vi "Initialize.vi"(8 "error in":errorcluster, 9 "Channels Amount":u8=1, 10 "InstanceName":string, 11 "Climate Chamber Cluster.lvclass":refnum<class "Climate Chamber Cluster.lvclass">) -> (0 "error out":errorcluster, 3 "Climate Chamber Cluster.lvclass out":refnum<class "Climate Chamber Cluster.lvclass">)   [LabVIEW 2023, in "Climate Chamber Cluster.lvclass"]
uses:
  Climate Chamber Cluster.lvclass
  Climate Chamber Cluster.lvclass/Climate Chamber Cluster.ctl
  310450b7-dc98-4d07-9383-43575356c6f4.vi
  702b615c-4a60-4ec7-b760-116075cb0d01.vi
  78d7c854-17cb-40e3-91c7-b55f38b06fec.vi
  34d8de8f-da75-496c-99f7-44cc67c60a3e.vi
  310450b7-dc98-4d07-9383-43575356c6f4.vi/4bc1c15b-36ab-481f-b8dd-c64075ce723a.vi
  702b615c-4a60-4ec7-b760-116075cb0d01.vi/4bc1c15b-36ab-481f-b8dd-c64075ce723a.vi
  78d7c854-17cb-40e3-91c7-b55f38b06fec.vi/4bc1c15b-36ab-481f-b8dd-c64075ce723a.vi
  34d8de8f-da75-496c-99f7-44cc67c60a3e.vi/4bc1c15b-36ab-481f-b8dd-c64075ce723a.vi
  <vilib>/ADAS Replay HIL/AdasHilServices/AdasHilServices Fill In Error Info Ex.vi
  Utilities/Utilities.lvlib
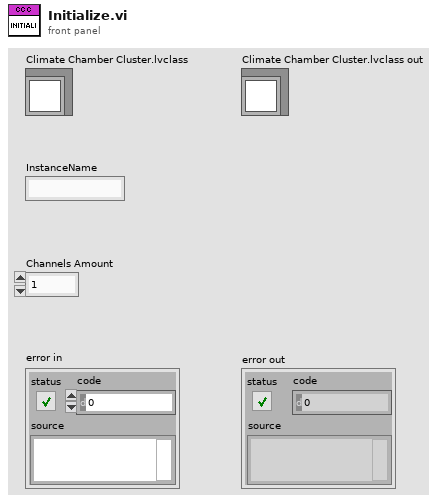
[diagram p1: front panel]
types:
  T1 = cluster{"OnOff.ACT":bool, "ErrorAcknowledge.ACT":bool}
  T2 = cluster{"OnOff.STS":i32, "Error.STS":i32, "Watchdog.STS":i32}
  T3 = cluster{"Temperature.SP":dbl, "TemperatureMIN.SP":dbl, "TemperatureMAX.SP":dbl, "TemperatureGrad.SP":dbl, "Humidity.SP":dbl, "HumidityMIN.SP":dbl, "HumidityMAX.SP":dbl, "HumidityGrad.SP":dbl}[]
  T4 = cluster{"Temperature.AV":dbl, "Humidity.AV":dbl}[]
  T5 = cluster{"Temperature.SP":dbl, "TemperatureMIN.SP":dbl, "TemperatureMAX.SP":dbl, "TemperatureGrad.SP":dbl, "Humidity.SP":dbl, "HumidityMIN.SP":dbl, "HumidityMAX.SP":dbl, "HumidityGrad.SP":dbl}
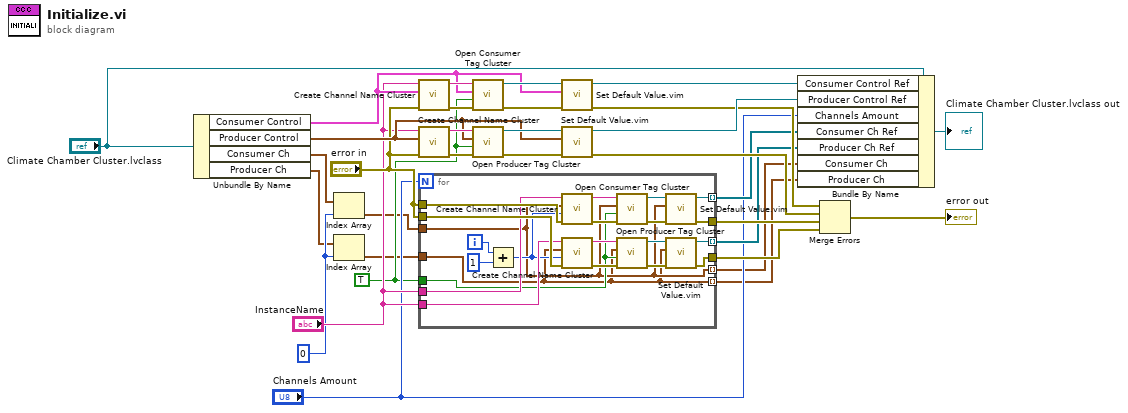
[diagram p0: block diagram]
diagram:
  w5 = 0 ("index")
  w8 = TRUE ("Create if not found? (T)")
  n1 = Unbundle By Name("Climate Chamber Cluster.lvclass") -> ("Consumer Control"=w18:T1, "Producer Control"=w19:T2, "Consumer Ch"=w7:T3, "Producer Ch"=w4:T4)
  n2 = Index Array(array=w7, index=w5) -> (element=w6:T5)
  n3 = Index Array(array=w4, index=w5) -> (element=w3:cluster{"Temperature.AV":dbl, "Humidity.AV":dbl})
  n4 = call "Create Channel Name Cluster.vi"("error in"="error in", "Cluster"=w18, "Instance Name"="InstanceName") -> ("error out"=w23:errorcluster, "Data Channel Name"=w32:string)  [unwired: 7 in]
  n5 = call "Create Channel Name Cluster.vi"("error in"="error in", "Cluster"=w19, "Instance Name"="InstanceName") -> ("error out"=w24:errorcluster, "Data Channel Name"=w31:string)  [unwired: 7 in]
  n6 = for {
    N: "Channels Amount" -> [_]
    tunnel: "error in" -> [w46]
    tunnel: "InstanceName" -> [w45]
    tunnel: "error in" -> [w44]
    tunnel: "InstanceName" -> [w43]
    tunnel: [w42] -> w15
    tunnel: [w41] -> w14
    tunnel: [w40] -> w12 mode=indexing
    tunnel: [w39] -> w11 mode=indexing
    tunnel: w6 -> [w34]
    tunnel: w3 -> [w33]
    tunnel: w8 -> [w38]
    tunnel: [w34] -> w2 mode=indexing
    tunnel: [w33] -> w1 mode=indexing
    i -> [w37]
    n7 = Add(x=w37, y=1) -> (x+y=w36:i32)
    n8 = call "Create Channel Name Cluster.vi"("error in"=w44, "Numeric"=w36, "Cluster"=w34, "Instance Name"=w43) -> ("error out"=w52:errorcluster, "Data Channel Name"=w47:string)  [unwired: 6 in]
    n9 = call "Create Channel Name Cluster.vi"("error in"=w46, "Numeric"=w36, "Cluster"=w33, "Instance Name"=w45) -> ("error out"=w54:errorcluster, "Data Channel Name"=w48:string)  [unwired: 6 in]
    n10 = call "Open Consumer Tag Cluster.vi"("error in"=w52, "Create if not found? (T)"=w38, "Cluster"=w34, "Channel Name"=w47) -> ("error out"=w51:errorcluster, "ADAS HIL Channel"=w50:refnum<k21>)  [unwired: 6 in]
    n11 = call "Open Producer Tag Cluster.vi"("error in"=w54, "Create if not found? (T)"=w38, "Cluster"=w33, "Channel Name"=w48) -> ("error out"=w53:errorcluster, "ADAS HIL Channel"=w49:refnum<k21>)  [unwired: 6 in]
    n12 = call "Set Default Value.vim"("error in"=w51, "Data in"=w34, "ADAS HIL Channel in"=w50) -> ("error out"=w41:errorcluster, "ADAS HIL Channel out"=w40:refnum<k21>)  [unwired: 7 in]
    n13 = call "Set Default Value.vim"("error in"=w53, "Data in"=w33, "ADAS HIL Channel in"=w49) -> ("error out"=w42:errorcluster, "ADAS HIL Channel out"=w39:refnum<k21>)  [unwired: 7 in]
  }
  n14 = call "Open Consumer Tag Cluster.vi"("error in"=w23, "Create if not found? (T)"=w8, "Cluster"=w18, "Channel Name"=w32) -> ("error out"=w28:errorcluster, "ADAS HIL Channel"=w30:refnum<k21>)  [unwired: 6 in]
  n15 = call "Open Producer Tag Cluster.vi"("error in"=w24, "Create if not found? (T)"=w8, "Cluster"=w19, "Channel Name"=w31) -> ("error out"=w27:errorcluster, "ADAS HIL Channel"=w26:refnum<k21>)  [unwired: 6 in]
  n16 = call "Set Default Value.vim"("error in"=w28, "Data in"=w18, "ADAS HIL Channel in"=w30) -> ("error out"=w22:errorcluster, "ADAS HIL Channel out"=w29:refnum<k21>)  [unwired: 7 in]
  n17 = call "Set Default Value.vim"("error in"=w27, "Data in"=w19, "ADAS HIL Channel in"=w26) -> ("error out"=w21:errorcluster, "ADAS HIL Channel out"=w25:refnum<k21>)  [unwired: 7 in]
  n18 = Bundle By Name(cluster="Climate Chamber Cluster.lvclass", "Consumer Control Ref"=w29, "Producer Control Ref"=w25, "Channels Amount"="Channels Amount", "Consumer Ch Ref"=w12, "Producer Ch Ref"=w11, "Consumer Ch"=w2, "Producer Ch"=w1) -> (→"Climate Chamber Cluster.lvclass out":refnum<class "Climate Chamber Cluster.lvclass">)
  n19 = Merge Errors(w22, w21, w14, w15) -> (→"error out":errorcluster)
